vi "Modbus_Master_global_ref_1.vi"(6 "Read:F/Wirte:T":bool, 8 "error in (no error) 2":errorcluster, 11 "Modbus Master In":refnum<class "Modbus Master.lvclass">) -> (0 "error out 2":errorcluster, 3 "Modbus Master out":refnum<class "Modbus Master.lvclass">)   [LabVIEW 2022 SP3]
uses:
  <vilib>/NI/Modbus Library/API/Master/Modbus Master.lvclass
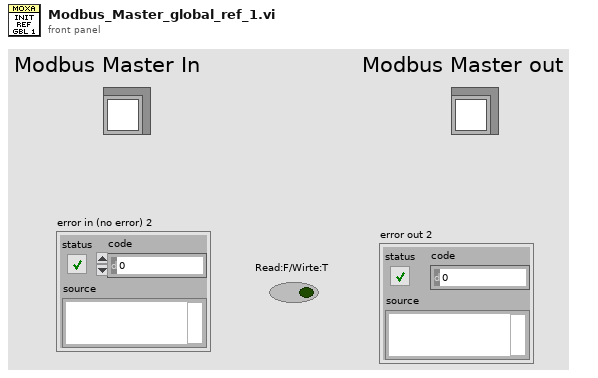
[diagram p1: front panel]
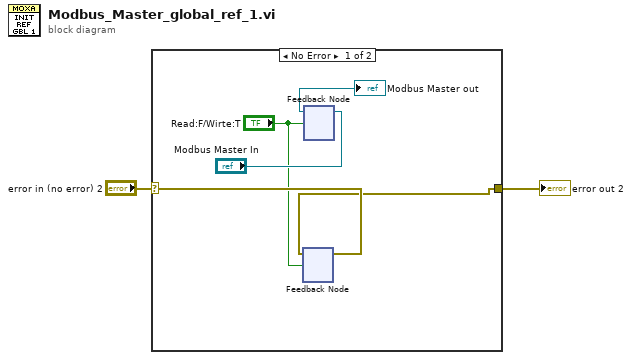
[diagram p0: block diagram]
diagram:
  n1 = case shown="No Error" "error in (no error) 2" {
    selector: "error in (no error) 2" -> [w5 w8]
    tunnel: [w4 w8] -> w1
    frame No Error {
      n2 = feedback #1() -> (w4:errorcluster)  [unwired: 1 in]
      n3 = feedback-in #1(w5, "Read:F/Wirte:T") -> ()
      n4 = feedback-in #2("Modbus Master In", "Read:F/Wirte:T") -> ()
      n5 = feedback #2() -> (→"Modbus Master out":refnum<class "Modbus Master.lvclass">)  [unwired: 1 in]
    }
    frame Error {
    }
  }
  "error out 2" <- w1
